vi "S2C_BldClearTable.vi"(8 "Error In":errorcluster) -> (0 "Error Out":errorcluster)   [LabVIEW 2015]
doc: "Clears the script table and associated controls."
uses:
  Globals/S2C_Globals.vi
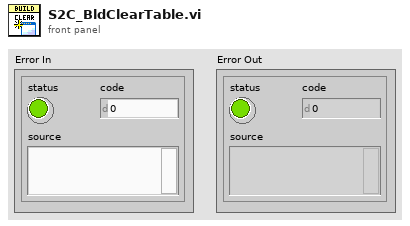
[diagram p1: front panel]
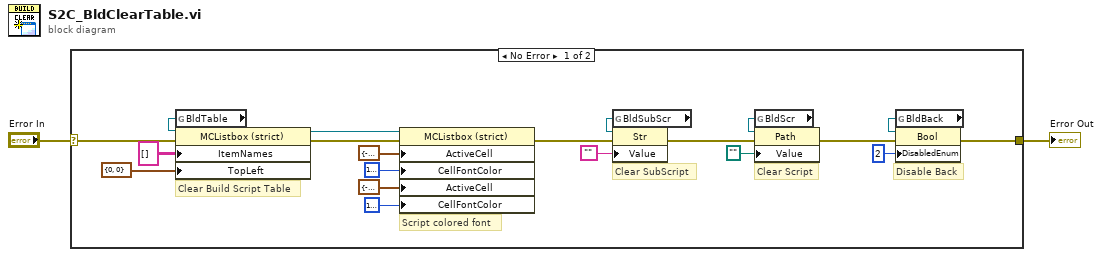
[diagram p0: block diagram]
diagram:
  n1 = case shown="No Error" "Error In" {
    selector: "Error In" -> [w18 w22]
    tunnel: [w13 w22] -> w1
    frame No Error {
      # "Script colored font"
      # "Disable Back"
      # "Clear Script"
      # "Clear SubScript"
      # "Clear Build Script Table"
      n2 = global read "S2C_Globals.vi" "BldTable"() -> (w21:refnum<vi>)
      n3 = property on="Property Node" class="MCListbox (strict)"(reference=w21, error in=w18, "ItemNames"=string[][] [] ("Item Names"), "TopLeft"=cluster{"Row":u32, "Column":u32} {"Row"=0, "Column"=0} ("Top Left Visible Cell")) -> (reference out=w4:refnum<vi>, error out=w5:errorcluster)
      n4 = property class="MCListbox (strict)"(reference=w4, error in=w5, "ActiveCell"=cluster{"Row":i32, "Column":i32} {"Row"=-2, "Column"=-2} ("Active Cell:Active Cell"), "CellFontColor"=u32 16777222, "ActiveCell"=cluster{"Row":i32, "Column":i32} {"Row"=-1, "Column"=-2} ("Active Cell:Active Cell"), "CellFontColor"=u32 16777226) -> (error out=w3:errorcluster)  [unwired: 1 out]
      n5 = global read "S2C_Globals.vi" "BldSubScr"() -> (w17:refnum<vi>)
      n6 = property class="Str"(reference=w17, error in=w3, "Value"="") -> (error out=w14:errorcluster)  [unwired: 1 out]
      n7 = global read "S2C_Globals.vi" "BldScr"() -> (w15:refnum<vi>)
      n8 = property class="Path"(reference=w15, error in=w14, "Value"=path "") -> (error out=w13:errorcluster)  [unwired: 1 out]
      n9 = global read "S2C_Globals.vi" "BldBack"() -> (w11:refnum<vi>)
      n10 = property class="Bool"(reference=w11, "DisabledEnum"=u8 2) -> ()  [unwired: 1 in, 2 out]
    }
    frame Error {
    }
  }
  "Error Out" <- w1
